vi "PIGraph3D_DLL_Functions.vi"(1 "ID in":i32=1 min=1 max=4 step=1, 2 "Window title":string, 3 "Function":T1(ring), 4 "Datastream":string, 5 "error in":errorcluster, 6 "Projections":u16(ring) items=["Plot only", "Plot + XY projection", "Plot + XZ projection", "Plot + YZ projection", "XY projection only", "XZ projection only", "YZ projection only"], 7 "Plot style":u16(ring) items=["Surface mode", "Hidden line mode", "Surface+line mode", "Wire mode"], 8 "Autoscale":bool=TRUE, 9 "ColourMap":u16(ring) items=["Spectrum", "Grayscale", "Blue_Red", "Red_Yellow", "Red_Green"], 10 "File path":string, 11 "No. of digits":i32[](array[numeric]), 12 "Orthogonal?":bool=TRUE, 13 "Show grid":bool=TRUE) -> (15 "ID out":i32=1 min=1 max=4 step=1, 19 "error out":errorcluster)   [LabVIEW 2026]
doc: "This VI calls a given function from GCSTranslator.dll. GCSTranslator.dll must be installed, and wxPIGraph3D.dll must be installed in PI\\GCSTranslator"
panel:
  out "autorange":i32
  # "This vi calls a given function from GCSTranslator.dll. GCSTranslator.dll must be installed, and\nwxPIGraph3D.dll must be installed in PI\\GCSTranslator."
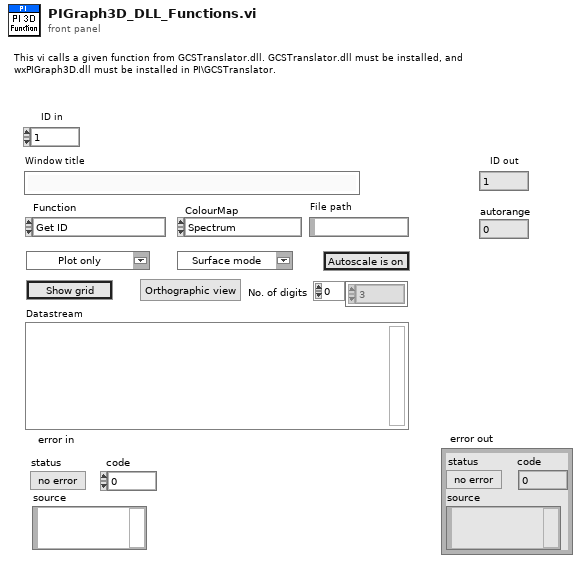
[diagram p1: front panel]
types:
  T1 = enum16{"Get ID", "Draw Data", "Clear Graph", "Projections", "Mode", "Colour", "Autoscale", "Show", "Close", "Save Image", "Set Digits", "Orthogonality", "Autoscale?", "Show Grid"}
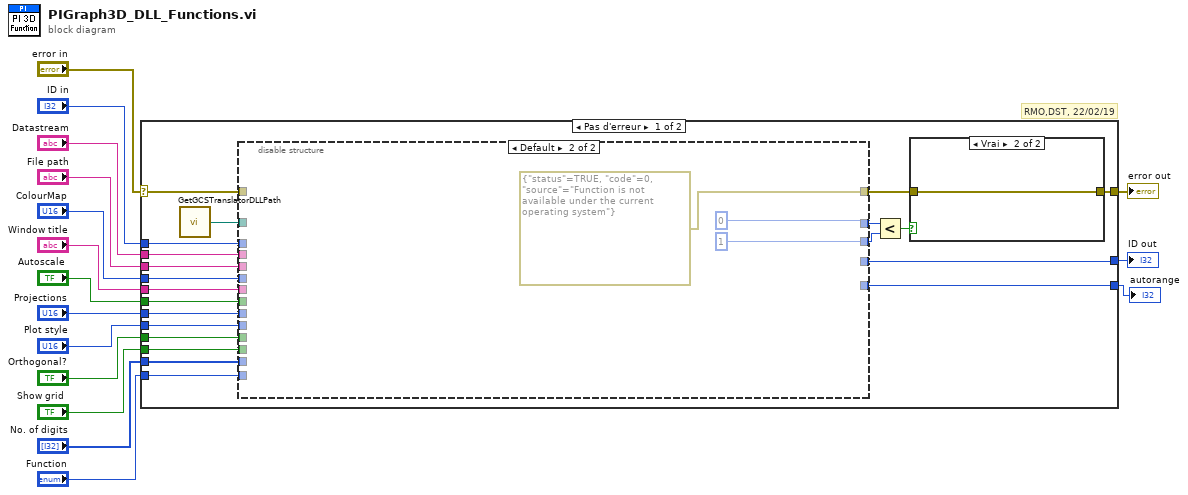
[diagram p0: block diagram]
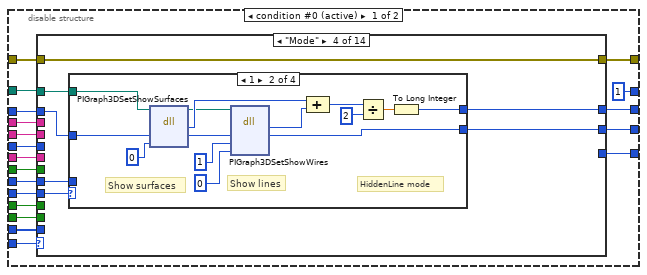
[diagram p2: hidden frame]
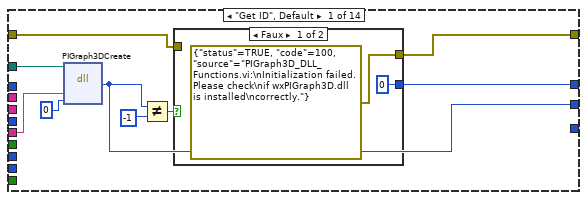
[diagram p3: hidden frame]
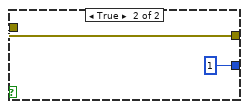
[diagram p4: hidden frame]
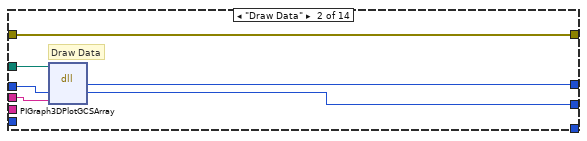
[diagram p5: hidden frame]
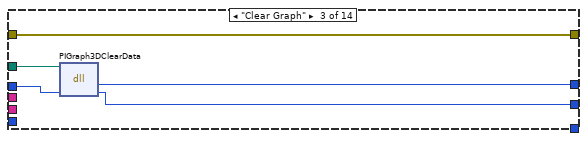
[diagram p6: hidden frame]
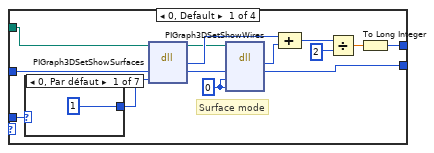
[diagram p7: hidden frame]
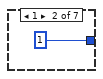
[diagram p8: hidden frame]
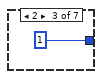
[diagram p9: hidden frame]
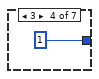
[diagram p10: hidden frame]
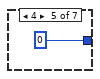
[diagram p11: hidden frame]
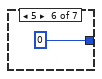
[diagram p12: hidden frame]
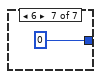
[diagram p13: hidden frame]
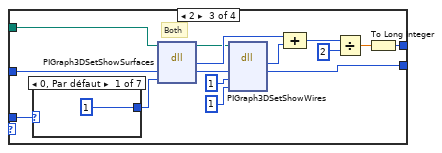
[diagram p14: hidden frame]
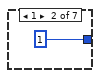
[diagram p15: hidden frame]
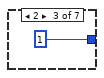
[diagram p16: hidden frame]
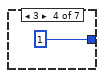
[diagram p17: hidden frame]
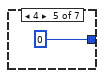
[diagram p18: hidden frame]
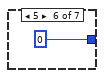
[diagram p19: hidden frame]
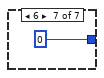
[diagram p20: hidden frame]
diagram:
  # "RMO,DST, 22/02/19"
  n1 = case shown="Pas d'erreur" "error in" {
    selector: "error in" -> [w34 w429]
    tunnel: "ID in" -> [w35 w428]
    tunnel: [w30 w429] -> w14
    tunnel: "Function" -> [w37 _]
    tunnel: [w36 w428] -> w12
    tunnel: "Projections" -> [w28 _]
    tunnel: "Plot style" -> [w27 _]
    tunnel: "Orthogonal?" -> [w26 _]
    tunnel: "Window title" -> [w25 _]
    tunnel: "Datastream" -> [w24 _]
    tunnel: "File path" -> [w23 _]
    tunnel: "ColourMap" -> [w22 _]
    tunnel: "Autoscale" -> [w21 _]
    tunnel: "Show grid" -> [w20 _]
    tunnel: "No. of digits" -> [w19 _]
    tunnel: [w17 0 ("autorange")] -> w1
    frame No Error {
      n2 = call "GetGCSTranslatorDLLPath.vi"() -> ("DLL path"=w18:path)  [unwired: 1 in]
      n3 = disable-structure shown="Default" {
        disable-tunnel: w37 -> [w56 _]
        disable-tunnel: [w55 w422] -> w36
        disable-tunnel: w35 -> [w54 _]
        disable-tunnel: w34 -> [w53 _]
        disable-tunnel: [1 ("y") 0 ("y")] -> w33
        disable-tunnel: [w51 w422] -> w32
        disable-tunnel: [w50 errorcluster {"status"=TRUE, "code"=0, "source"="Function is not available under the current operating system"} ("error IO")] -> w29
        disable-tunnel: w28 -> [w49 _]
        disable-tunnel: w27 -> [w48 _]
        disable-tunnel: w26 -> [w47 _]
        disable-tunnel: w25 -> [w46 _]
        disable-tunnel: w24 -> [w45 _]
        disable-tunnel: w23 -> [w44 _]
        disable-tunnel: w22 -> [w43 _]
        disable-tunnel: w21 -> [w42 _]
        disable-tunnel: w20 -> [w41 _]
        disable-tunnel: [w40 w422] -> w17
        disable-tunnel: w19 -> [w39 _]
        disable-tunnel: w18 -> [w38 _]
        frame condition #0 (active) {
          n4 = case shown="\"Mode\"" w56 {
            tunnel: [w60 w75 w79 w86 w164 w177 w195 w204 w230 w392 w400 w407 w415 w420] -> w55
            tunnel: w54 -> [_ w74 w80 w87 w165 w190 w197 w209 w231 w393 w401 w408 w416 w421]
            tunnel: w53 -> [w64 w73 w78 w85 w162 w189 w194 w206 w229 w391 w398 w406 w414 w419]
            tunnel: [w62 w73 w78 w85 w162 w189 w194 w206 w229 w391 w398 w406 w414 w419] -> w50
            tunnel: [w59 w72 w77 w84 w161 w170 w193 w202 w227 w389 w397 w405 w413 w418] -> w51
            tunnel: w49 -> [_ _ _ w82 _ _ _ _ w226 _ _ _ _ _]
            tunnel: w48 -> [_ _ _ w83 _ _ _ _ w225 _ _ _ _ _]
            tunnel: w47 -> [_ _ _ _ _ _ _ _ _ _ _ w403 _ _]
            tunnel: w46 -> [w58 _ _ _ _ _ _ _ _ _ _ _ _ _]
            tunnel: w45 -> [_ w71 _ _ _ _ _ _ _ _ _ _ _ _]
            tunnel: w44 -> [_ _ _ _ w160 _ _ _ _ _ _ _ _ _]
            tunnel: w43 -> [_ _ _ _ _ _ w192 _ _ _ _ _ _ _]
            tunnel: w42 -> [_ _ _ _ _ _ _ w201 _ _ _ _ _ _]
            tunnel: w41 -> [_ _ _ _ _ _ _ _ _ w388 _ _ _ _]
            tunnel: [_ _ _ _ _ _ _ _ _ _ _ _ w412 _] -> w40
            tunnel: w39 -> [_ _ _ _ _ w169 _ _ _ _ _ _ _ _]
            tunnel: w38 -> [w57 w70 w76 w81 w159 w168 w191 w200 w224 w387 w396 w402 w411 w417]
            frame "Get ID", Default {
              n5 = dll-call lib="T:/Entwicklung/HostSoftware/LabVIEW/GCSDrivers/source/GCS2LabVIEW/Low Level/GCSTranslator.dll" fn="PIGraph3DCreate"(path in=w57, "title"=w58, "bshow"=0) -> ("return type"=w60:i32)  [unwired: 4 in, 2 out]
              n6 = Not Equal?(x=w60, y=-1) -> (x != y?=w63:bool)
              n7 = case shown="Faux" w63 {
                tunnel: w64 -> [_ w69]
                tunnel: [errorcluster {"status"=TRUE, "code"=100, "source"="PIGraph3D_DLL_Functions.vi:\nInitialization failed. Please check\nif wxPIGraph3D.dll is installed\ncorrectly."} ("error IO") w69] -> w62
                tunnel: [0 1] -> w59
                frame False {
                }
                frame True {
                }
              }
            }
            frame "Draw Data" {
              # "Draw Data"
              n8 = dll-call lib="T:/Entwicklung/HostSoftware/LabVIEW/GCSDrivers/source/GCS2LabVIEW/Low Level/GCSTranslator.dll" fn="PIGraph3DPlotGCSArray"(path in=w70, "ID"=w74, "GCSArray"=w71) -> ("return type"=w72:i32, "ID"=w75:i32)  [unwired: 3 in, 2 out]
            }
            frame "Clear Graph" {
              n9 = dll-call lib="T:/Entwicklung/HostSoftware/LabVIEW/GCSDrivers/source/GCS2LabVIEW/Low Level/GCSTranslator.dll" fn="PIGraph3DClearData"(path in=w76, "ID"=w80) -> ("return type"=w77:i32, "ID"=w79:i32)  [unwired: 2 in, 2 out]
            }
            frame "Mode" {
              n10 = case shown="1" w83 {
                tunnel: w87 -> [w100 w121 w137 w157]
                tunnel: [w98 w118 w134 w154] -> w86
                tunnel: [w91 w111 w127 w147] -> w84
                tunnel: w82 -> [w90 _ w126 _]
                tunnel: w81 -> [w89 w110 w124 w146]
                frame 0, Default {
                  w97 = 0 ("bShowSurfaces")
                  # "Surface mode"
                  n11 = case shown="0, Par défaut" w90 {
                    tunnel: [1 ("bShowSurfaces") 1 ("bShowSurfaces") 1 ("bShowSurfaces") 1 ("bShowSurfaces") 0 ("bShowSurfaces") 0 ("bShowSurfaces") 0 ("bShowSurfaces")] -> w101
                    frame 0, Default {
                    }
                    frame 1 {
                    }
                    frame 2 {
                    }
                    frame 3 {
                    }
                    frame 4 {
                    }
                    frame 5 {
                    }
                    frame 6 {
                    }
                  }
                  n12 = dll-call lib="T:/Entwicklung/HostSoftware/LabVIEW/GCSDrivers/source/GCS2LabVIEW/Low Level/GCSTranslator.dll" fn="PIGraph3DSetShowSurfaces"(path in=w89, "ID"=w100, "bShowSurfaces"=w101) -> (path out=w88:path, "return type"=w93:i32, "ID"=w99:i32)  [unwired: 3 in, 1 out]
                  n13 = dll-call lib="T:/Entwicklung/HostSoftware/LabVIEW/GCSDrivers/source/GCS2LabVIEW/Low Level/GCSTranslator.dll" fn="PIGraph3DSetShowWires"(path in=w88, "ID"=w99, "bShowWires"=w97, "bShowHiddenWires"=w97) -> ("return type"=w92:i32, "ID"=w98:i32)  [unwired: 4 in, 2 out]
                  n14 = Compound Arithmetic op=ADD(w93, w92) -> (w96:i32)
                  n15 = Divide(x=w96, y=2) -> (x/y=w94:dbl)
                  n16 = To Long Integer(number=w94) -> (32bit integer=w91:i32)
                }
                frame 1 {
                  # "Show lines"
                  # "Show surfaces"
                  # "HiddenLine mode"
                  n17 = dll-call lib="T:/Entwicklung/HostSoftware/LabVIEW/GCSDrivers/source/GCS2LabVIEW/Low Level/GCSTranslator.dll" fn="PIGraph3DSetShowSurfaces"(path in=w110, "ID"=w121, "bShowSurfaces"=0) -> (path out=w109:path, "return type"=w113:i32, "ID"=w120:i32)  [unwired: 3 in, 1 out]
                  n18 = dll-call lib="T:/Entwicklung/HostSoftware/LabVIEW/GCSDrivers/source/GCS2LabVIEW/Low Level/GCSTranslator.dll" fn="PIGraph3DSetShowWires"(path in=w109, "ID"=w120, "bShowWires"=1 ("bShowSurfaces"), "bShowHiddenWires"=0) -> ("return type"=w112:i32, "ID"=w118:i32)  [unwired: 4 in, 2 out]
                  n19 = Compound Arithmetic op=ADD(w113, w112) -> (w116:i32)
                  n20 = Divide(x=w116, y=2) -> (x/y=w114:dbl)
                  n21 = To Long Integer(number=w114) -> (32bit integer=w111:i32)
                }
                frame 2 {
                  # "Both"
                  n22 = case shown="0, Par défaut" w126 {
                    tunnel: [1 ("bShowSurfaces") 1 ("bShowSurfaces") 1 ("bShowSurfaces") 1 ("bShowSurfaces") 0 ("bShowSurfaces") 0 ("bShowSurfaces") 0 ("bShowSurfaces")] -> w125
                    frame 0, Default {
                    }
                    frame 1 {
                    }
                    frame 2 {
                    }
                    frame 3 {
                    }
                    frame 4 {
                    }
                    frame 5 {
                    }
                    frame 6 {
                    }
                  }
                  n23 = dll-call lib="T:/Entwicklung/HostSoftware/LabVIEW/GCSDrivers/source/GCS2LabVIEW/Low Level/GCSTranslator.dll" fn="PIGraph3DSetShowSurfaces"(path in=w124, "ID"=w137, "bShowSurfaces"=w125) -> (path out=w123:path, "return type"=w129:i32, "ID"=w136:i32)  [unwired: 3 in, 1 out]
                  n24 = dll-call lib="T:/Entwicklung/HostSoftware/LabVIEW/GCSDrivers/source/GCS2LabVIEW/Low Level/GCSTranslator.dll" fn="PIGraph3DSetShowWires"(path in=w123, "ID"=w136, "bShowWires"=1 ("bShowSurfaces"), "bShowHiddenWires"=1) -> ("return type"=w128:i32, "ID"=w134:i32)  [unwired: 4 in, 2 out]
                  n25 = Compound Arithmetic op=ADD(w129, w128) -> (w132:i32)
                  n26 = Divide(x=w132, y=2) -> (x/y=w130:dbl)
                  n27 = To Long Integer(number=w130) -> (32bit integer=w127:i32)
                }
                frame 3 {
                  # "Wire mode"
                  n28 = dll-call lib="T:/Entwicklung/HostSoftware/LabVIEW/GCSDrivers/source/GCS2LabVIEW/Low Level/GCSTranslator.dll" fn="PIGraph3DSetShowSurfaces"(path in=w146, "ID"=w157, "bShowSurfaces"=0) -> (path out=w145:path, "return type"=w149:i32, "ID"=w156:i32)  [unwired: 3 in, 1 out]
                  n29 = dll-call lib="T:/Entwicklung/HostSoftware/LabVIEW/GCSDrivers/source/GCS2LabVIEW/Low Level/GCSTranslator.dll" fn="PIGraph3DSetShowWires"(path in=w145, "ID"=w156, "bShowWires"=1 ("bShowSurfaces"), "bShowHiddenWires"=1) -> ("return type"=w148:i32, "ID"=w154:i32)  [unwired: 4 in, 2 out]
                  n30 = Compound Arithmetic op=ADD(w149, w148) -> (w152:i32)
                  n31 = Divide(x=w152, y=2) -> (x/y=w150:dbl)
                  n32 = To Long Integer(number=w150) -> (32bit integer=w147:i32)
                }
              }
            }
            frame "Save Image" {
              n33 = dll-call lib="T:/Entwicklung/HostSoftware/LabVIEW/GCSDrivers/source/GCS2LabVIEW/Low Level/GCSTranslator.dll" fn="PIGraph3DSaveToImageFile"(path in=w159, "ID"=w165, "szFilename"=w160, "type"=2) -> ("return type"=w161:i32, "ID"=w164:i32)  [unwired: 4 in, 2 out]
            }
            frame "Set Digits" {
              n34 = Index Array(array=w169, index=0 ("axis")) -> (element=w180:i32)
              n35 = Index Array(array=w169, index=1 ("axis")) -> (element=w179:i32)
              n36 = Index Array(array=w169, index=2 ("axis")) -> (element=w178:i32)
              n37 = dll-call lib="T:/Entwicklung/HostSoftware/LabVIEW/GCSDrivers/source/GCS2LabVIEW/Low Level/GCSTranslator.dll" fn="PIGraph3DSetTickDigits"(path in=w168, "ID"=w190, "axis"=1, "digits"=w180) -> (path out=w167:path, "return type"=w174:i32, "ID"=w184:i32)  [unwired: 4 in, 1 out]
              n38 = dll-call lib="T:/Entwicklung/HostSoftware/LabVIEW/GCSDrivers/source/GCS2LabVIEW/Low Level/GCSTranslator.dll" fn="PIGraph3DSetTickDigits"(path in=w167, "ID"=w184, "axis"=2, "digits"=w179) -> (path out=w166:path, "return type"=w173:i32, "ID"=w181:i32)  [unwired: 4 in, 1 out]
              n39 = dll-call lib="T:/Entwicklung/HostSoftware/LabVIEW/GCSDrivers/source/GCS2LabVIEW/Low Level/GCSTranslator.dll" fn="PIGraph3DSetTickDigits"(path in=w166, "ID"=w181, "axis"=3, "digits"=w178) -> ("return type"=w172:i32, "ID"=w177:i32)  [unwired: 4 in, 2 out]
              n40 = Compound Arithmetic op=ADD(w174, w173, w172) -> (w176:i32)
              n41 = Divide(x=w176, y=3) -> (x/y=w171:dbl)
              n42 = To Long Integer(number=w171) -> (32bit integer=w170:i32)
            }
            frame "Colour" {
              n43 = property on="ColourMap" class="MDér (strict)"() -> ("Strings []"=w198:string[])  [unwired: 2 in, 2 out]
              n44 = Index Array(array=w198, index=w192) -> (element=w196:string)
              n45 = dll-call lib="T:/Entwicklung/HostSoftware/LabVIEW/GCSDrivers/source/GCS2LabVIEW/Low Level/GCSTranslator.dll" fn="PIGraph3DSelectColourMap"(path in=w191, "ID"=w197, "szColourMapName"=w196) -> ("return type"=w193:i32, "ID"=w195:i32)  [unwired: 2 in, 3 out]
            }
            frame "Autoscale" {
              n46 = Boolean To (0,1)(Boolean=w201) -> (0, 1=w208:i16)
              n47 = To Long Integer(number=w208) -> (32bit integer=w207:i32)
              n48 = dll-call lib="T:/Entwicklung/HostSoftware/LabVIEW/GCSDrivers/source/GCS2LabVIEW/Low Level/GCSTranslator.dll" fn="PIGraph3DSetAutoRange"(path in=w200, "ID"=w209, "bAutoRange"=w207) -> (path out=w199:path, "return type"=w203:i32, "ID"=w205:i32)  [unwired: 3 in, 1 out]
              n49 = case shown="Faux" w201 {
                tunnel: w205 -> [w218 w223]
                tunnel: [w217 w223] -> w204
                tunnel: w203 -> [w213 w222]
                tunnel: [w211 w222] -> w202
                tunnel: w199 -> [w210 _]
                frame False {
                  n50 = dll-call lib="T:/Entwicklung/HostSoftware/LabVIEW/GCSDrivers/source/GCS2LabVIEW/Low Level/GCSTranslator.dll" fn="PIGraph3DSetRange"(path in=w210, "ID"=w218, "axis"=3, "dmin"=0.0, "dmax"=10.0 ("dmin")) -> ("return type"=w212:i32, "ID"=w217:i32)  [unwired: 5 in, 2 out]
                  n51 = Compound Arithmetic op=ADD(w213, w212) -> (w216:i32)
                  n52 = Divide(x=w216, y=2) -> (x/y=w214:dbl)
                  n53 = To Long Integer(number=w214) -> (32bit integer=w211:i32)
                }
                frame True {
                }
              }
            }
            frame "Projections" {
              n54 = case shown="1" w226 {
                tunnel: w231 -> [w245 w268 w288 w309 w328 w348 w369]
                tunnel: [w250 w274 w294 w314 w334 w354 w374] -> w230
                tunnel: [w237 w261 w281 w301 w321 w341 w361] -> w228
                tunnel: w225 -> [w236 _ _ _ _ _ _]
                tunnel: w224 -> [w235 w260 w280 w300 w320 w340 w360]
                frame 0, Default {
                  # "Plot"
                  # "Plot only"
                  n55 = case shown="0, Par défaut" w236 {
                    tunnel: [1 ("bShowSurfaces") 0 ("bShowSurfaces") 1 ("bShowSurfaces") 0 ("bShowSurfaces")] -> w246
                    frame 0, Default {
                    }
                    frame 1 {
                    }
                    frame 2 {
                    }
                    frame 3 {
                    }
                  }
                  n56 = dll-call lib="T:/Entwicklung/HostSoftware/LabVIEW/GCSDrivers/source/GCS2LabVIEW/Low Level/GCSTranslator.dll" fn="PIGraph3DSetShowSurfaces"(path in=w235, "ID"=w245, "bShowSurfaces"=w246) -> (path out=w234:path, "return type"=w241:i32, "ID"=w244:i32)  [unwired: 3 in, 1 out]
                  n57 = dll-call lib="T:/Entwicklung/HostSoftware/LabVIEW/GCSDrivers/source/GCS2LabVIEW/Low Level/GCSTranslator.dll" fn="PIGraph3DSetDrawXYProjection"(path in=w234, "ID"=w244, "bShow"=0) -> (path out=w233:path, "return type"=w240:i32, "ID"=w252:i32)  [unwired: 3 in, 1 out]
                  n58 = dll-call lib="T:/Entwicklung/HostSoftware/LabVIEW/GCSDrivers/source/GCS2LabVIEW/Low Level/GCSTranslator.dll" fn="PIGraph3DSetDrawXZProjection"(path in=w233, "ID"=w252, "bShow"=0) -> (path out=w232:path, "return type"=w239:i32, "ID"=w251:i32)  [unwired: 3 in, 1 out]
                  n59 = dll-call lib="T:/Entwicklung/HostSoftware/LabVIEW/GCSDrivers/source/GCS2LabVIEW/Low Level/GCSTranslator.dll" fn="PIGraph3DSetDrawYZProjection"(path in=w232, "ID"=w251, "bShow"=0) -> ("return type"=w238:i32, "ID"=w250:i32)  [unwired: 3 in, 2 out]
                  n60 = Compound Arithmetic op=ADD(w241, w240, w239, w238) -> (w243:i32)
                  n61 = Divide(x=w243, y=4) -> (x/y=w237:dbl)
                }
                frame 1 {
                  # "Plot"
                  # "YZ"
                  # "XZ"
                  # "XY"
                  # "Plot + XY projection"
                  n62 = dll-call lib="T:/Entwicklung/HostSoftware/LabVIEW/GCSDrivers/source/GCS2LabVIEW/Low Level/GCSTranslator.dll" fn="PIGraph3DSetShowSurfaces"(path in=w260, "ID"=w268, "bShowSurfaces"=1) -> (path out=w259:path, "return type"=w265:i32, "ID"=w269:i32)  [unwired: 3 in, 1 out]
                  n63 = dll-call lib="T:/Entwicklung/HostSoftware/LabVIEW/GCSDrivers/source/GCS2LabVIEW/Low Level/GCSTranslator.dll" fn="PIGraph3DSetDrawXYProjection"(path in=w259, "ID"=w269, "bShow"=1) -> (path out=w258:path, "return type"=w264:i32, "ID"=w276:i32)  [unwired: 3 in, 1 out]
                  n64 = dll-call lib="T:/Entwicklung/HostSoftware/LabVIEW/GCSDrivers/source/GCS2LabVIEW/Low Level/GCSTranslator.dll" fn="PIGraph3DSetDrawXZProjection"(path in=w258, "ID"=w276, "bShow"=0) -> (path out=w257:path, "return type"=w263:i32, "ID"=w275:i32)  [unwired: 3 in, 1 out]
                  n65 = dll-call lib="T:/Entwicklung/HostSoftware/LabVIEW/GCSDrivers/source/GCS2LabVIEW/Low Level/GCSTranslator.dll" fn="PIGraph3DSetDrawYZProjection"(path in=w257, "ID"=w275, "bShow"=0) -> ("return type"=w262:i32, "ID"=w274:i32)  [unwired: 3 in, 2 out]
                  n66 = Compound Arithmetic op=ADD(w265, w264, w263, w262) -> (w267:i32)
                  n67 = Divide(x=w267, y=4) -> (x/y=w261:dbl)
                }
                frame 2 {
                  # "Plot"
                  # "YZ"
                  # "XZ"
                  # "XY"
                  # "Plot + XZ projection"
                  n68 = dll-call lib="T:/Entwicklung/HostSoftware/LabVIEW/GCSDrivers/source/GCS2LabVIEW/Low Level/GCSTranslator.dll" fn="PIGraph3DSetShowSurfaces"(path in=w280, "ID"=w288, "bShowSurfaces"=1) -> (path out=w279:path, "return type"=w285:i32, "ID"=w289:i32)  [unwired: 3 in, 1 out]
                  n69 = dll-call lib="T:/Entwicklung/HostSoftware/LabVIEW/GCSDrivers/source/GCS2LabVIEW/Low Level/GCSTranslator.dll" fn="PIGraph3DSetDrawXYProjection"(path in=w279, "ID"=w289, "bShow"=0) -> (path out=w278:path, "return type"=w284:i32, "ID"=w296:i32)  [unwired: 3 in, 1 out]
                  n70 = dll-call lib="T:/Entwicklung/HostSoftware/LabVIEW/GCSDrivers/source/GCS2LabVIEW/Low Level/GCSTranslator.dll" fn="PIGraph3DSetDrawXZProjection"(path in=w278, "ID"=w296, "bShow"=1) -> (path out=w277:path, "return type"=w283:i32, "ID"=w295:i32)  [unwired: 3 in, 1 out]
                  n71 = dll-call lib="T:/Entwicklung/HostSoftware/LabVIEW/GCSDrivers/source/GCS2LabVIEW/Low Level/GCSTranslator.dll" fn="PIGraph3DSetDrawYZProjection"(path in=w277, "ID"=w295, "bShow"=0) -> ("return type"=w282:i32, "ID"=w294:i32)  [unwired: 3 in, 2 out]
                  n72 = Compound Arithmetic op=ADD(w285, w284, w283, w282) -> (w287:i32)
                  n73 = Divide(x=w287, y=4) -> (x/y=w281:dbl)
                }
                frame 3 {
                  # "Plot"
                  # "YZ"
                  # "XZ"
                  # "XY"
                  # "Plot + YZ projection"
                  n74 = dll-call lib="T:/Entwicklung/HostSoftware/LabVIEW/GCSDrivers/source/GCS2LabVIEW/Low Level/GCSTranslator.dll" fn="PIGraph3DSetShowSurfaces"(path in=w300, "ID"=w309, "bShowSurfaces"=1) -> (path out=w299:path, "return type"=w305:i32, "ID"=w308:i32)  [unwired: 3 in, 1 out]
                  n75 = dll-call lib="T:/Entwicklung/HostSoftware/LabVIEW/GCSDrivers/source/GCS2LabVIEW/Low Level/GCSTranslator.dll" fn="PIGraph3DSetDrawXYProjection"(path in=w299, "ID"=w308, "bShow"=0) -> (path out=w298:path, "return type"=w304:i32, "ID"=w316:i32)  [unwired: 3 in, 1 out]
                  n76 = dll-call lib="T:/Entwicklung/HostSoftware/LabVIEW/GCSDrivers/source/GCS2LabVIEW/Low Level/GCSTranslator.dll" fn="PIGraph3DSetDrawXZProjection"(path in=w298, "ID"=w316, "bShow"=0) -> (path out=w297:path, "return type"=w303:i32, "ID"=w315:i32)  [unwired: 3 in, 1 out]
                  n77 = dll-call lib="T:/Entwicklung/HostSoftware/LabVIEW/GCSDrivers/source/GCS2LabVIEW/Low Level/GCSTranslator.dll" fn="PIGraph3DSetDrawYZProjection"(path in=w297, "ID"=w315, "bShow"=1) -> ("return type"=w302:i32, "ID"=w314:i32)  [unwired: 3 in, 2 out]
                  n78 = Compound Arithmetic op=ADD(w305, w304, w303, w302) -> (w307:i32)
                  n79 = Divide(x=w307, y=4) -> (x/y=w301:dbl)
                }
                frame 4 {
                  # "Plot"
                  # "YZ"
                  # "XZ"
                  # "XY"
                  # "XY projection only"
                  n80 = dll-call lib="T:/Entwicklung/HostSoftware/LabVIEW/GCSDrivers/source/GCS2LabVIEW/Low Level/GCSTranslator.dll" fn="PIGraph3DSetShowSurfaces"(path in=w320, "ID"=w328, "bShowSurfaces"=0) -> (path out=w319:path, "return type"=w325:i32, "ID"=w329:i32)  [unwired: 3 in, 1 out]
                  n81 = dll-call lib="T:/Entwicklung/HostSoftware/LabVIEW/GCSDrivers/source/GCS2LabVIEW/Low Level/GCSTranslator.dll" fn="PIGraph3DSetDrawXYProjection"(path in=w319, "ID"=w329, "bShow"=1) -> (path out=w318:path, "return type"=w324:i32, "ID"=w336:i32)  [unwired: 3 in, 1 out]
                  n82 = dll-call lib="T:/Entwicklung/HostSoftware/LabVIEW/GCSDrivers/source/GCS2LabVIEW/Low Level/GCSTranslator.dll" fn="PIGraph3DSetDrawXZProjection"(path in=w318, "ID"=w336, "bShow"=0) -> (path out=w317:path, "return type"=w323:i32, "ID"=w335:i32)  [unwired: 3 in, 1 out]
                  n83 = dll-call lib="T:/Entwicklung/HostSoftware/LabVIEW/GCSDrivers/source/GCS2LabVIEW/Low Level/GCSTranslator.dll" fn="PIGraph3DSetDrawYZProjection"(path in=w317, "ID"=w335, "bShow"=0) -> ("return type"=w322:i32, "ID"=w334:i32)  [unwired: 3 in, 2 out]
                  n84 = Compound Arithmetic op=ADD(w325, w324, w323, w322) -> (w327:i32)
                  n85 = Divide(x=w327, y=4) -> (x/y=w321:dbl)
                }
                frame 5 {
                  # "Plot"
                  # "YZ"
                  # "XZ"
                  # "XY"
                  # "Plot only"
                  n86 = dll-call lib="T:/Entwicklung/HostSoftware/LabVIEW/GCSDrivers/source/GCS2LabVIEW/Low Level/GCSTranslator.dll" fn="PIGraph3DSetShowSurfaces"(path in=w340, "ID"=w348, "bShowSurfaces"=0) -> (path out=w339:path, "return type"=w345:i32, "ID"=w349:i32)  [unwired: 3 in, 1 out]
                  n87 = dll-call lib="T:/Entwicklung/HostSoftware/LabVIEW/GCSDrivers/source/GCS2LabVIEW/Low Level/GCSTranslator.dll" fn="PIGraph3DSetDrawXYProjection"(path in=w339, "ID"=w349, "bShow"=0) -> (path out=w338:path, "return type"=w344:i32, "ID"=w356:i32)  [unwired: 3 in, 1 out]
                  n88 = dll-call lib="T:/Entwicklung/HostSoftware/LabVIEW/GCSDrivers/source/GCS2LabVIEW/Low Level/GCSTranslator.dll" fn="PIGraph3DSetDrawXZProjection"(path in=w338, "ID"=w356, "bShow"=1) -> (path out=w337:path, "return type"=w343:i32, "ID"=w355:i32)  [unwired: 3 in, 1 out]
                  n89 = dll-call lib="T:/Entwicklung/HostSoftware/LabVIEW/GCSDrivers/source/GCS2LabVIEW/Low Level/GCSTranslator.dll" fn="PIGraph3DSetDrawYZProjection"(path in=w337, "ID"=w355, "bShow"=0) -> ("return type"=w342:i32, "ID"=w354:i32)  [unwired: 3 in, 2 out]
                  n90 = Compound Arithmetic op=ADD(w345, w344, w343, w342) -> (w347:i32)
                  n91 = Divide(x=w347, y=4) -> (x/y=w341:dbl)
                }
                frame 6 {
                  # "Plot"
                  # "YZ"
                  # "XZ"
                  # "XY"
                  # "YZ projection only"
                  n92 = dll-call lib="T:/Entwicklung/HostSoftware/LabVIEW/GCSDrivers/source/GCS2LabVIEW/Low Level/GCSTranslator.dll" fn="PIGraph3DSetShowSurfaces"(path in=w360, "ID"=w369, "bShowSurfaces"=0) -> (path out=w359:path, "return type"=w367:i32, "ID"=w368:i32)  [unwired: 3 in, 1 out]
                  n93 = dll-call lib="T:/Entwicklung/HostSoftware/LabVIEW/GCSDrivers/source/GCS2LabVIEW/Low Level/GCSTranslator.dll" fn="PIGraph3DSetDrawXYProjection"(path in=w359, "ID"=w368, "bShow"=0) -> (path out=w358:path, "return type"=w366:i32, "ID"=w376:i32)  [unwired: 3 in, 1 out]
                  n94 = dll-call lib="T:/Entwicklung/HostSoftware/LabVIEW/GCSDrivers/source/GCS2LabVIEW/Low Level/GCSTranslator.dll" fn="PIGraph3DSetDrawXZProjection"(path in=w358, "ID"=w376, "bShow"=0) -> (path out=w357:path, "return type"=w365:i32, "ID"=w375:i32)  [unwired: 3 in, 1 out]
                  n95 = dll-call lib="T:/Entwicklung/HostSoftware/LabVIEW/GCSDrivers/source/GCS2LabVIEW/Low Level/GCSTranslator.dll" fn="PIGraph3DSetDrawYZProjection"(path in=w357, "ID"=w375, "bShow"=1) -> ("return type"=w364:i32, "ID"=w374:i32)  [unwired: 3 in, 2 out]
                  n96 = Compound Arithmetic op=ADD(w367, w366, w365, w364) -> (w363:i32)
                  n97 = Divide(x=w363, y=4) -> (x/y=w361:dbl)
                }
              }
              n98 = To Long Integer(number=w228) -> (32bit integer=w227:i32)
            }
            frame "Show Grid" {
              n99 = case shown="Vrai" w388 {
                tunnel: [0 ("bShow") 1 ("bShow")] -> w386
                frame False {
                  # "Grid oFF"
                }
                frame True {
                  # "Grid on"
                }
              }
              n100 = dll-call lib="T:/Entwicklung/HostSoftware/LabVIEW/GCSDrivers/source/GCS2LabVIEW/Low Level/GCSTranslator.dll" fn="PIGraph3DSetDrawXYGrid"(path in=w387, "ID"=w393, "bShow"=w386) -> (path out=w378:path, "return type"=w381:i32, "ID"=w385:i32)  [unwired: 3 in, 1 out]
              n101 = dll-call lib="T:/Entwicklung/HostSoftware/LabVIEW/GCSDrivers/source/GCS2LabVIEW/Low Level/GCSTranslator.dll" fn="PIGraph3DSetDrawXZGrid"(path in=w378, "ID"=w385, "bShow"=w386) -> (path out=w377:path, "return type"=w380:i32, "ID"=w384:i32)  [unwired: 3 in, 1 out]
              n102 = dll-call lib="T:/Entwicklung/HostSoftware/LabVIEW/GCSDrivers/source/GCS2LabVIEW/Low Level/GCSTranslator.dll" fn="PIGraph3DSetDrawYZGrid"(path in=w377, "ID"=w384, "bShow"=w386) -> ("return type"=w379:i32, "ID"=w392:i32)  [unwired: 3 in, 2 out]
              n103 = Compound Arithmetic op=ADD(w381, w380, w379) -> (w383:i32)
              n104 = Divide(x=w383, y=3) -> (x/y=w390:dbl)
              n105 = To Long Integer(number=w390) -> (32bit integer=w389:i32)
            }
            frame "Show" {
              n106 = dll-call lib="T:/Entwicklung/HostSoftware/LabVIEW/GCSDrivers/source/GCS2LabVIEW/Low Level/GCSTranslator.dll" fn="PIGraph3DShow"(path in=w396, "ID"=w401, "bShow"=1) -> ("return type"=w397:i32, "ID"=w400:i32)  [unwired: 3 in, 2 out]
            }
            frame "Orthogonality" {
              n107 = case shown="Faux" w403 {
                tunnel: [2 1] -> w404
                frame False {
                }
                frame True {
                }
              }
              n108 = dll-call lib="T:/Entwicklung/HostSoftware/LabVIEW/GCSDrivers/source/GCS2LabVIEW/Low Level/GCSTranslator.dll" fn="PIGraph3DSetProjection"(path in=w402, "ID"=w408, "projection"=w404) -> ("return type"=w405:i32, "ID"=w407:i32)  [unwired: 3 in, 2 out]
            }
            frame "Autoscale?" {
              n109 = dll-call lib="T:/Entwicklung/HostSoftware/LabVIEW/GCSDrivers/source/GCS2LabVIEW/Low Level/GCSTranslator.dll" fn="PIGraph3DGetAutoRange"(path in=w411, "ID"=w416) -> ("return type"=w413:i32, "ID"=w415:i32, "autorange"=w412:i32)  [unwired: 2 in, 3 out]
            }
            frame "Close" {
              n110 = dll-call lib="T:/Entwicklung/HostSoftware/LabVIEW/GCSDrivers/source/GCS2LabVIEW/Low Level/GCSTranslator.dll" fn="PIGraph3DClose"(path in=w417, "ID"=w421) -> ("return type"=w418:i32, "ID"=w420:i32)  [unwired: 2 in, 2 out]
            }
          }
        }
        frame condition #1 {
          w422 = 1
        }
      }
      n111 = Less?(x=w33, y=w32) -> (x < y?=w31:bool)
      n112 = case shown="Vrai" w31 {
        tunnel: [errorcluster {"status"=TRUE, "code"=100, "source"="PIGraph3D_DLL_Functions.vi:\nFunction call failed."} ("error IO") w426] -> w30
        tunnel: w29 -> [_ w426]
        frame False {
        }
        frame True {
        }
      }
    }
    frame Error {
    }
  }
  "error out" <- w14
  "ID out" <- w12
  "autorange" <- w1
